vi "Traccia_I_V_DIFF.vi"() -> ()   [LabVIEW 2014]
doc: "Traccia_I_V\nUtilizza Vu_fisso e traccia una curva Vout vs Vin\nGrafica la corrente vs Tensione\n2011/09, mod 2013/9\nFM & ADL"
uses:
  <vilib>/Utility/file.llb/Write To Spreadsheet File (DBL).vi
panel:
  in  "Fondo Scala AI1":dbl(ring)=10.0 items=["10"=10.0, "5"=5.0, "0.5"=0.5, "0.05"=0.05]
  in  "Scala Asse Y":enum8{"Lineare", "Logaritmica"}(ring)
  in  "R (Ohm)":dbl=220.0 min=0.0 max=100000.0 step=10.0 format="%_4g"
  in  "Fondo Scala AI0":dbl(ring)=10.0 items=["10"=10.0, "5"=5.0, "0.5"=0.5, "0.05"=0.05]
  in  "SALVA I DATI SU FILE":bool=TRUE caption="ON\nOFF"
  out "N. misura":i16=20
  out "Corrente in funzione della tensione":cluster{dbl[], dbl[]}(graph)={[0.0, 0.26281609786184207, 0.4530736019736842, 0.5160361842105263, 0.5493845086348683, 0.5738949424342104, 0.5926192434210527, 0.6054109272203947, 0.6161518297697368, 0.6301398026315788, 0.6393914473684208, 0.6486430921052628, 0.6530119243421053, 0.6622635690789473, 0.6707095497532896, 0.6807668585526314, 0.6900185032894735, 0.6971705386513158, 0.7035901521381573, 0.7080078125], [0.0, 0.000341796875, 0.0732421875, 0.2734375, 0.5032470703125, 0.74189453125, 0.986328125, 1.2366943359375, 1.489111328125, 1.73828125, 1.9921875, 2.24609375, 2.5048828125, 2.7587890625, 3.0135009765625, 3.2666015625, 3.5205078125, 3.776513671875, 4.033251953125, 4.2919921875]}
  out "Vin (V)":dbl=5.0 format="%_4g"
  out "V (V)":dbl=4.2919921875 format="%_4f"
  in  "Numero misure":i16=20 min=0 max=1000 step=1
  in  "Vmax(V)x":dbl=5.0 min=0.0 max=8.0 step=0.1 format="%_4g"
  in  "Vmin(V)":dbl min=0.0 max=8.0 step=0.1 format="%_4g"
  # "1) Scegliere il fondo scala deidue ingressi analogici, la resistenza R (in Ohm) e la tipologia di scala sull'asse Y."
  # "Collegare il CB 22 (Analog Output 0) all'ingresso Vin (vedi figura) e i due capi dell'elemento da misurare ai CB68  e CB34 (vedi figura). \nV  e' la tensione ai capi del dispositivo sotto misura, I la corrente che vi scorre.\nLa terra del circuito DEVE essere in comune alla terra della scheda  (CB29)."
  # "2) Selezionare il valore minimo e massimo della tensione di ingresso Vin ed il numero di valori \n(equispaziati  tra gli estremi)"
  # "Durante la misura gli indicatori mostrano i valori di Vin e Vout ed il numero progressivo della misura"
  # "Sul grafico viene mostrata la corrente I in funzione della tensione V"
  # "NO\nSI"
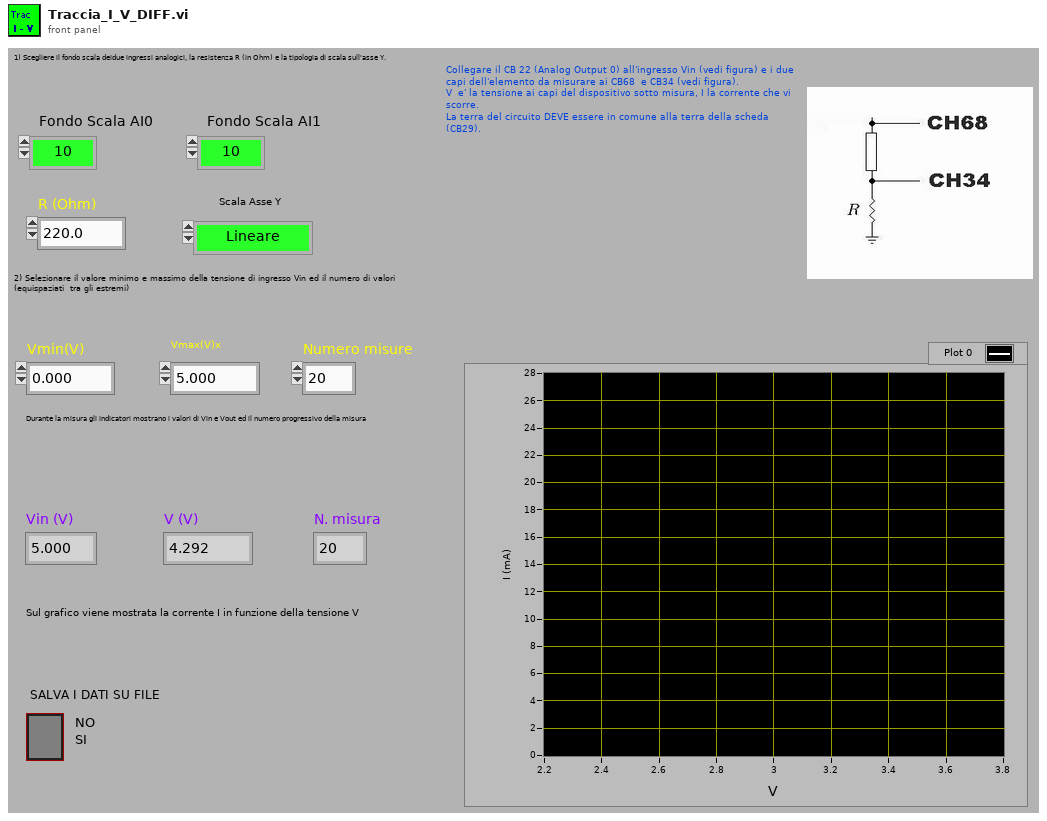
[diagram p1: front panel]
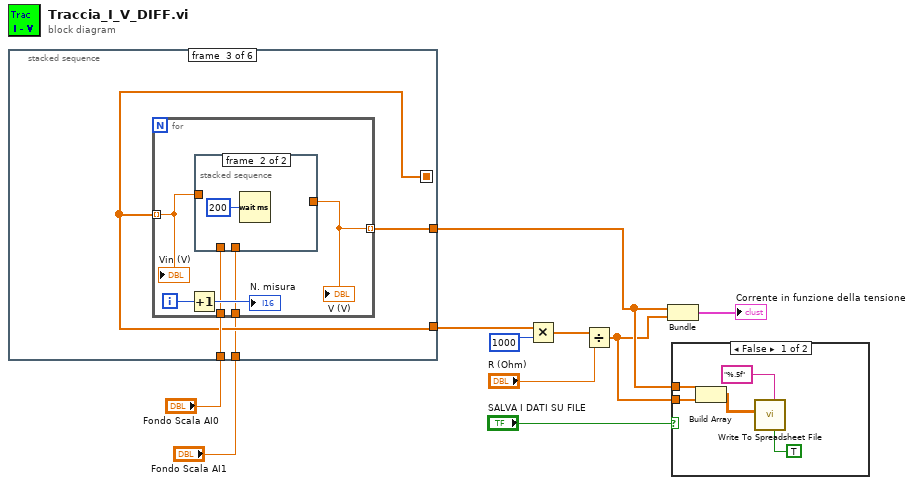
[diagram p0: block diagram]
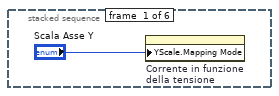
[diagram p3: hidden frame]
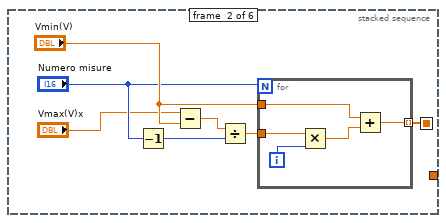
[diagram p4: hidden frame]
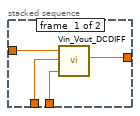
[diagram p5: hidden frame]
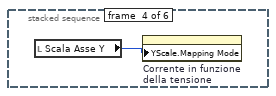
[diagram p6: hidden frame]
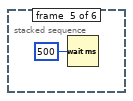
[diagram p7: hidden frame]
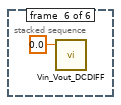
[diagram p8: hidden frame]
diagram:
  n1 = stacked-sequence {
    seq-local: [_ w14 _ _ _ _] -> [_ _ w25 _ _ _]
    tunnel: [_ _ w25 _ _ _] -> w3
    tunnel: [_ _ w26 _ _ _] -> w9
    tunnel: "Fondo Scala AI0" -> [_ _ w27 _ _ _]
    tunnel: "Fondo Scala AI1" -> [_ _ w24 _ _ _]
    frame #0 {
      n2 = property on="Corrente in funzione della tensione" class="XYGraph (strict)"("YScale.Mapping Mode"="Scala Asse Y") -> ()  [unwired: 2 in, 2 out]
    }
    frame #1 {
      n3 = Decrement(x="Numero misure") -> (x-1=w17:i16)
      n4 = Subtract(x="Vmax(V)x", y="Vmin(V)") -> (x-y=w18:dbl)
      n5 = Divide(x=w18, y=w17) -> (x/y=w16:dbl)
      n6 = for {
        N: "Numero misure" -> [_]
        tunnel: "Vmin(V)" -> [w23]
        tunnel: [w22] -> w14 mode=indexing
        tunnel: w16 -> [w21]
        i -> [w20]
        n7 = Multiply(x=w21, y=w20) -> (x*y=w19:dbl)
        n8 = Add(x=w23, y=w19) -> (x+y=w22:dbl)
      }
    }
    frame #2 {
      n9 = for {
        tunnel: w25 -> [w33] mode=indexing
        tunnel: [w32] -> w26 mode=indexing
        tunnel: w27 -> [w29]
        tunnel: w24 -> [w28]
        i -> [w31]
        n10 = Increment(x=w31) -> (x+1=→"N. misura":i32)
        n11 = stacked-sequence {
          tunnel: w33 -> [w36 _]
          tunnel: [w37 _] -> w32
          tunnel: w29 -> [w35 _]
          tunnel: w28 -> [w34 _]
          frame #0 {
            n12 = call "Vin_Vout_DCDIFF.vi"("V in volt"=w36, "Fondo Scala AI0 (68-34)"=w35, "Fondo Scala AI1 (33)"=w34) -> ("sd 0"=w37:dbl)  [unwired: 3 out]
          }
          frame #1 {
            n13 = Wait (ms)(milliseconds to wait=u32 200) -> ()  [unwired: 1 out]
          }
        }
        "V (V)" <- w32
        "Vin (V)" <- w33
      }
    }
    frame #3 {
      n14 = local read "Scala Asse Y"() -> (w39:enum8{"Lineare", "Logaritmica"})
      n15 = property on="Corrente in funzione della tensione" class="XYGraph (strict)"("YScale.Mapping Mode"=w39) -> ()  [unwired: 2 in, 2 out]
    }
    frame #4 {
      n16 = Wait (ms)(milliseconds to wait=u32 500) -> ()  [unwired: 1 out]
    }
    frame #5 {
      n17 = call "Vin_Vout_DCDIFF.vi"("V in volt"=0.0 ("V_in (Volt)")) -> ()  [unwired: 2 in, 4 out]
    }
  }
  n18 = Multiply(x=w3, y=1000) -> (x*y=w2:dbl[])
  n19 = Divide(x=w2, y="R (Ohm)") -> (x/y=w6:dbl[])
  n20 = Bundle(w9, w6) -> (→"Corrente in funzione della tensione":cluster{dbl[], dbl[]})  [unwired: 1 out]
  n21 = case shown="False" "SALVA I DATI SU FILE" {
    tunnel: w6 -> [w46 _]
    tunnel: w9 -> [w45 _]
    frame False {
      n22 = Build Array(w45, w46) -> (w44:dbl[][])
      n23 = call-poly <vilib>:"Write To Spreadsheet File.vi"("transpose? (no:F)"=TRUE, "format (%.3f)"="%.5f", "2D data"=w44) -> ()  [unwired: 3 in, 3 out]
    }
    frame True {
    }
  }
